vi "Call@USERCallVISample.vi__Parameter.vi"(1 "ParamterIn":string) -> (0 "ParamterOut":string)   [LabVIEW 2020]
uses:
  MainFrame/Global.vi
panel:
  in  "Parameters":string(combo)
  in  "VI":string(combo)
  in  "Confirm":bool
  # "Call@USERCallVISample.vi $Parameter1,$Parameter2"
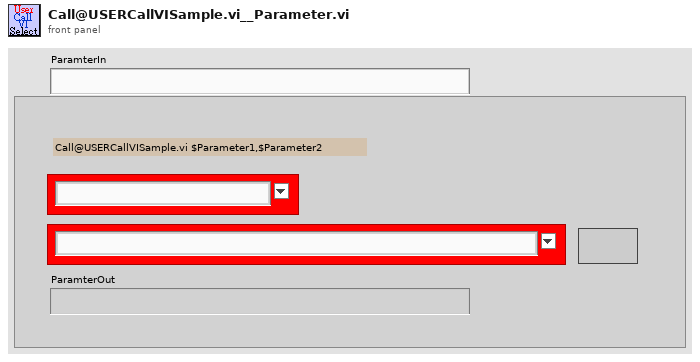
[diagram p1: front panel]
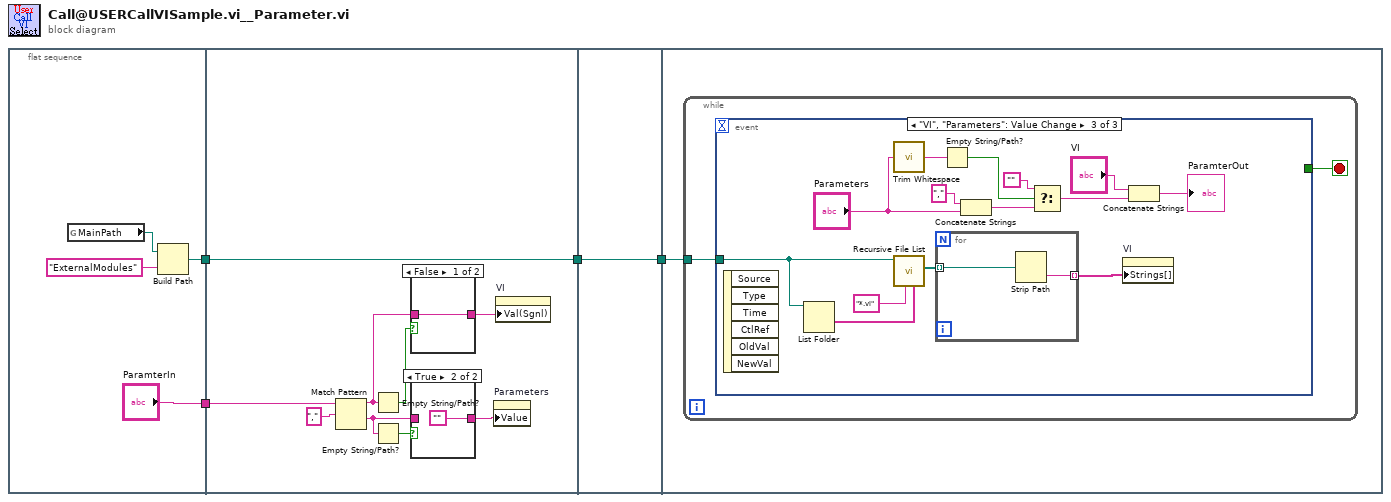
[diagram p0: block diagram]
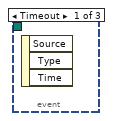
[diagram p4: hidden frame]
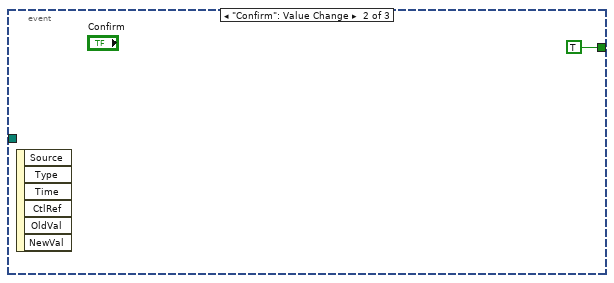
[diagram p5: hidden frame]
diagram:
  n1 = flat-sequence {
    tunnel: [w7] -> w2
    tunnel: ["ParamterIn"] -> w1
    tunnel: [w15] -> w3
    tunnel: w2 -> [w15]
    tunnel: w1 -> [w9]
    tunnel: [w22] -> w4
    tunnel: w3 -> [w22]
    tunnel: w4 -> [w23]
    frame #0 {
      n2 = global read "Global.vi" "MainPath"() -> (w6:path)
      n3 = Build Path(base path=w6, name or relative path="ExternalModules") -> (appended path=w7:path)
    }
    frame #1 {
      n4 = Match Pattern(string=w9, regular expression=",") -> (before substring=w13:string, after substring=w12:string)  [unwired: 1 in, 2 out]
      n5 = Empty String/Path?(string/path=w13) -> (empty?=w17:bool)
      n6 = Empty String/Path?(string/path=w12) -> (empty?=w16:bool)
      n7 = case shown="False" w17 {
        tunnel: w13 -> [w20 w21]
        tunnel: [w20 w21] -> w10
        frame False {
        }
        frame True {
        }
      }
      n8 = case shown="True" w16 {
        tunnel: [w18 ""] -> w11
        tunnel: w12 -> [w18 _]
        frame False {
        }
        frame True {
        }
      }
      n9 = property on="Parameters" class="CmbBox"("Value"=w11) -> ()  [unwired: 2 in, 2 out]
      n10 = property on="VI" class="CmbBox"("Val(Sgnl)"=w10) -> ()  [unwired: 2 in, 2 out]
    }
    frame #2 {
    }
    frame #3 {
      n11 = while {
        tunnel: w23 -> [w24]
        stop <- w25 stop-if-true
        n12 = event shown="[2] \"VI\", \"Parameters\": Value Change" {
          selector: _ -> [_ _ _]
          dyn-events: _ -> [_ _ _]
          timeout: _ -> [_ _ _]
          tunnel: [_ TRUE _] -> w25
          tunnel: w24 -> [_ _ w28]
          event Timeout {
            n13 = event-data() -> ()  [unwired: 1 in, 3 out]
          }
          event "Confirm": Value Change {
            n14 = event-data() -> ()  [unwired: 1 in, 6 out]
          }
          event "VI", "Parameters": Value Change {
            n15 = event-data() -> ()  [unwired: 1 in, 6 out]
            n16 = List Folder(path=w28) -> (folder names=w27:string[])  [unwired: 3 in, 3 out]
            n17 = call <vilib>:"Trim Whitespace.vi"("string"="Parameters") -> ("trimmed string"=w34:string)  [unwired: 1 in]
            n18 = call <vilib>:"Recursive File List.vi"("Folders to Exclude"=w27, "pattern"="*.vi", "Folder Path"=w28) -> ("All Files in Dir"=w38:path[])  [unwired: 4 in, 4 out]
            n19 = for {
              tunnel: w38 -> [w42] mode=indexing
              tunnel: [w41] -> w30 mode=indexing
              n20 = Strip Path(path=w42) -> (name=w41:string)  [unwired: 1 out]
            }
            n21 = Empty String/Path?(string/path=w34) -> (empty?=w35:bool)
            n22 = Concatenate Strings("," ("string"), "Parameters") -> (w33:string)
            n23 = Select(t="", s=w35, f=w33) -> (s? t:f=w29:string)
            n24 = property on="VI" class="CmbBox"("Strings[]"=w30) -> ()  [unwired: 2 in, 2 out]
            n25 = Concatenate Strings("VI", w29) -> (→"ParamterOut":string)
          }
        }
      }
    }
  }
